vi "ex_getChanNamesFromDDT.vi"(8 "error in (no error)":errorcluster, 9 "file params":T3 {"Flags"."time preference" items=["Absolute", "Relative"]; "Flags"."x_columns" items=["None", "One", "Multiple"]; "origin time" format="%<%X\n%x>T"}, 10 "append info in":T1, 11 "Express Wave Attributes in":T2[](array[typedef]) {"dX" format="%.2f"; "X0" format="%<%X\n%x>T"; "Timestamp" format="%<%X\n%x>T"; "Start Timestamp" format="%<%X\n%x>T"}) -> (0 "error out":errorcluster, 1 "channels match":bool, 2 "channel names":string[](array[string]), 3 "Express Wave Attributes out":T2[](array[typedef]) {"dX" format="%.2f"; "X0" format="%<%X\n%x>T"; "Timestamp" format="%<%X\n%x>T"; "Start Timestamp" format="%<%X\n%x>T"}, 5 "error code":i32)   [LabVIEW 2017]
uses:
  <vilib>/express/express output/ExFileWriteBlock.llb/ex_WriteFileParams.ctl
  <vilib>/express/express input/ExFileReadBlock.llb/ex_ReadFileParams.ctl
  <vilib>/express/express shared/transition.llb/ex_WaveformAttribsPlus.ctl
  <vilib>/Platform/express/TDMExpress.llb/ex_appendInfoTDM.ctl
panel:
  out "dT":dbl[](array[numeric])
  out "Array 4":dbl[](array[numeric])
  out "channel types":string[](array[string])
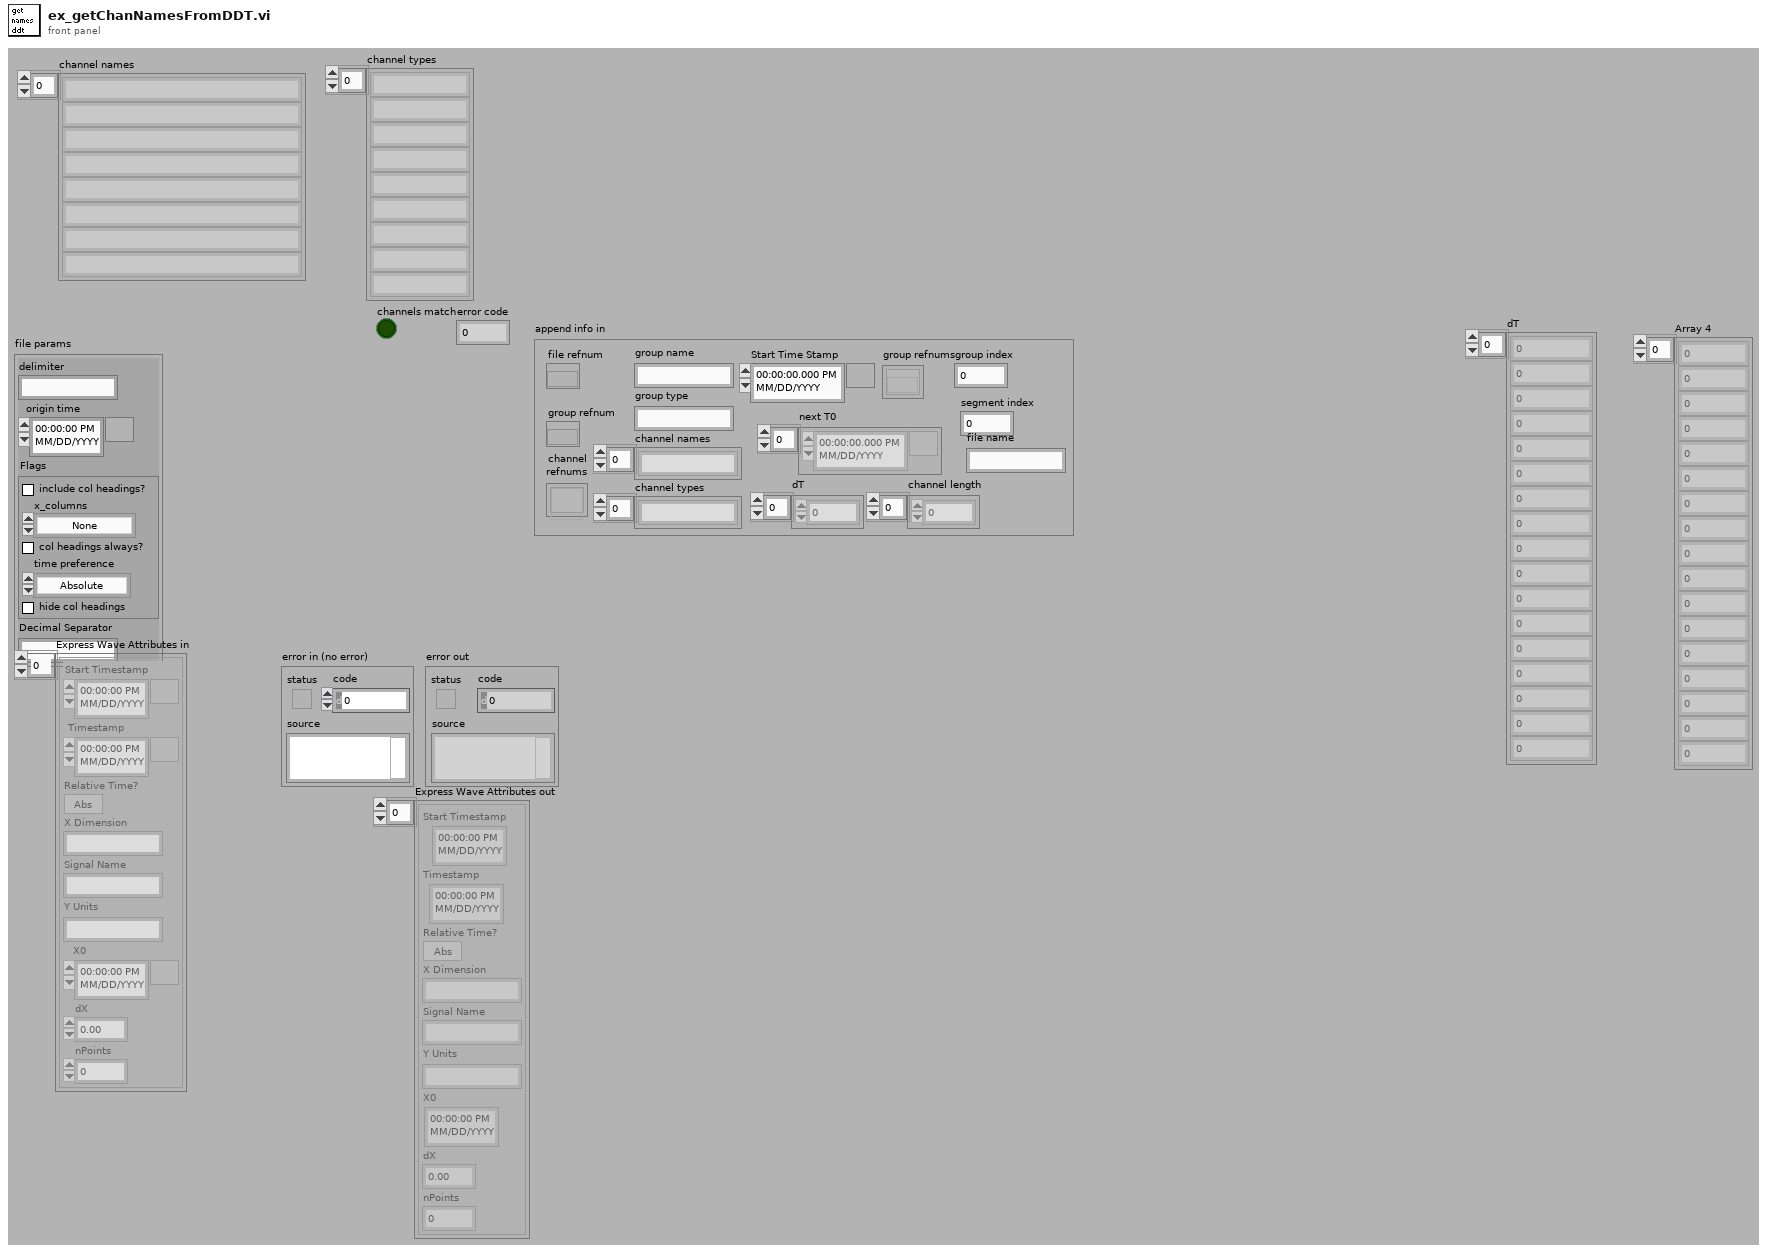
[diagram p1: front panel]
types:
  T1 = typedef "ex_appendInfoTDM.ctl" = cluster{"channel\nrefnums":refnum<k20>[], "channel names":string[], "channel types":string[], "file refnum":refnum<k20>, "group refnum":refnum<k20>, "group name":string, "group type":string, "next T0":timestamp[], "dT":dbl[], "Start Time Stamp":timestamp, "channel length":u32[], "group index":u32, "group refnums":refnum<k20>[], "file name":string, "segment index":u32}
  T2 = typedef "ex_WaveformAttribsPlus.ctl" = cluster{"Start Timestamp":timestamp, "Timestamp":timestamp, "Relative Time?":bool, "X Dimension":string, "Signal Name":string, "Y Units":string, "X0":timestamp, "dX":dbl, "nPoints":i32}
  T3 = typedef "ex_WriteFileParams.ctl" = cluster{"delimiter":string, "origin time":timestamp, "Flags":T4, "Decimal Separator":string}
  T4 = typedef "ex_ReadFileParams.ctl" = cluster{"include col headings?":bool, "x_columns":u16, "col headings always?":bool, "time preference":u16, "hide col headings":bool}
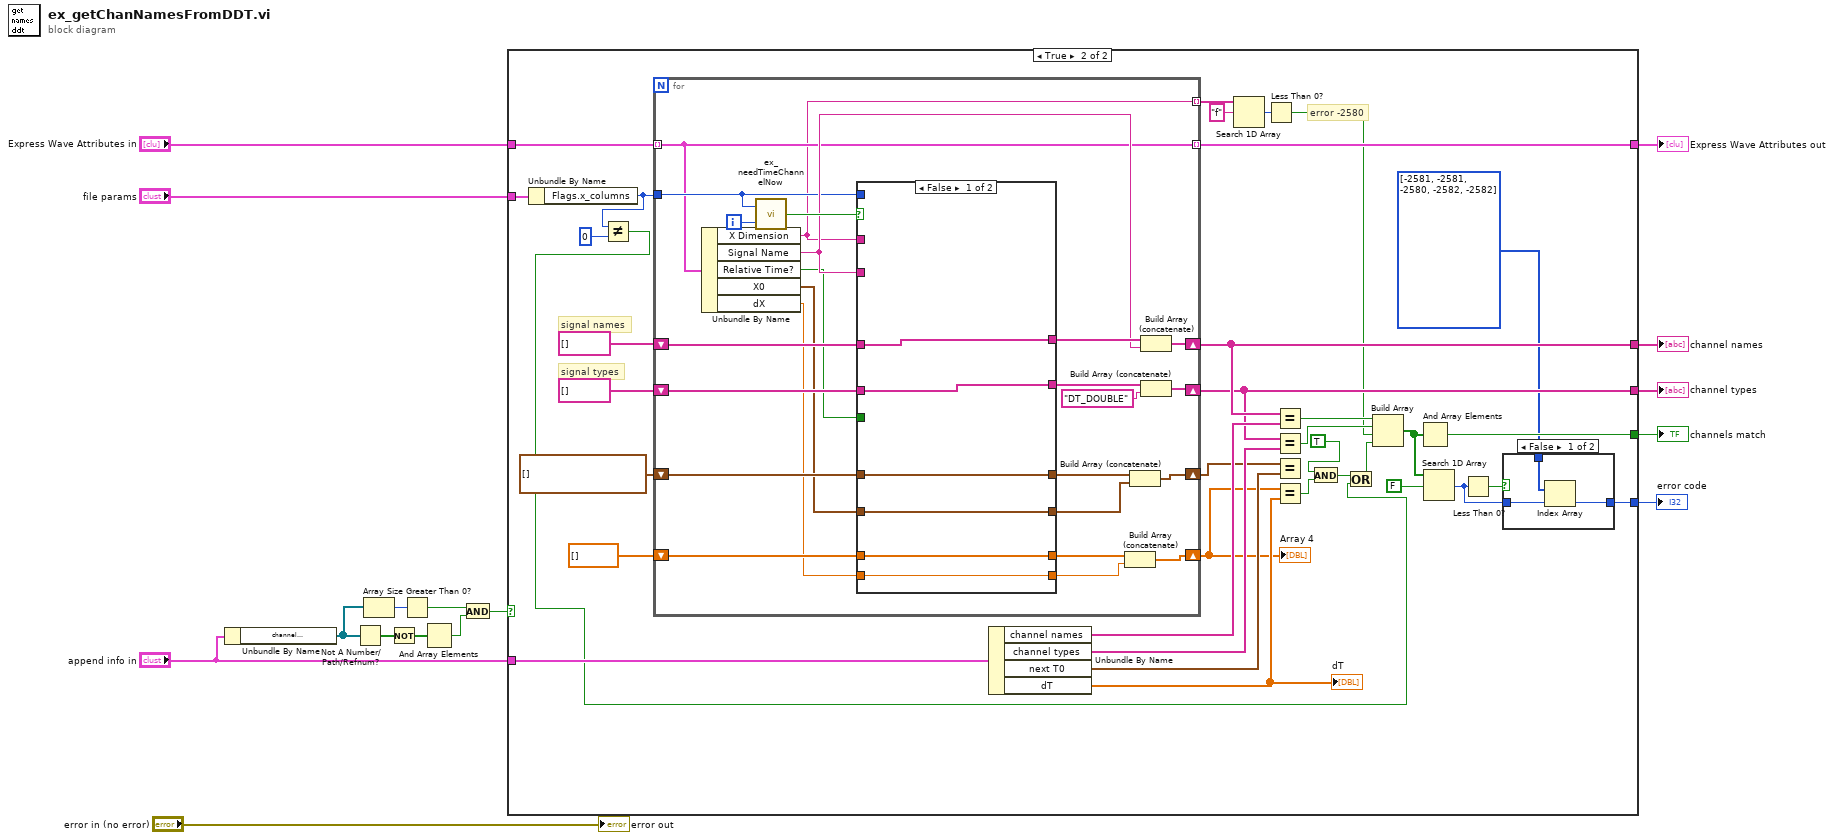
[diagram p0: block diagram]
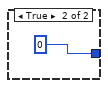
[diagram p3: hidden frame]
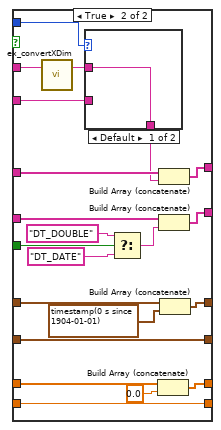
[diagram p4: hidden frame]
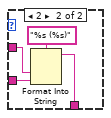
[diagram p5: hidden frame]
diagram:
  n1 = Unbundle By Name("append info in") -> ("channel\nrefnums"=w6:refnum<k20>[])
  n2 = Not A Number/Path/Refnum?(number/path/refnum=w6) -> (NaN/Path/Refnum?=w12:bool[])
  n3 = Array Size(array=w6) -> (size(s)=w5:i32)
  n4 = Not(x=w12) -> (.not. x?=w11:bool[])
  n5 = Greater Than 0?(x=w5) -> (x > 0?=w3:bool)
  n6 = And Array Elements(Boolean array=w11) -> (logical AND=w4:bool)
  n7 = And(x=w3, y=w4) -> (x .and. y?=w2:bool)
  n8 = case shown="True" w2 {
    tunnel: "file params" -> [_ w53]
    tunnel: "Express Wave Attributes in" -> [w17 w51]
    tunnel: [w17 w49] -> w13
    tunnel: [_ w48] -> w10
    tunnel: [_ w36] -> w9
    tunnel: "append info in" -> [_ w44]
    tunnel: [_ w43] -> w7
    tunnel: [_ w32] -> w1
    frame False {
    }
    frame True {
      # "error -2580"
      # "signal types"
      # "signal names"
      n9 = Unbundle By Name(w53) -> ("Flags.x_columns"=w21:u16)
      n10 = Not Equal?(x=w21, y=u16 0) -> (x != y?=w19:bool)
      n11 = for {
        tunnel: w51 -> [w69] mode=indexing
        tunnel: w21 -> [w75]
        shift-right: [w78] -> w48
        shift-left: string[] [] -> [w79]
        shift-right: [w72] -> w43
        shift-left: string[] [] -> [w74]
        tunnel: [w69] -> w49 mode=indexing
        tunnel: [w68] -> w42 mode=indexing
        shift-right: [w65] -> w26
        shift-left: timestamp[] [] -> [w67]
        shift-right: [w59] -> w25
        shift-left: dbl[] [] -> [w62]
        i -> [w81]
        n12 = Unbundle By Name(w69) -> ("X Dimension"=w68:string, "Signal Name"=w76:string, "Relative Time?"=w73:bool, "X0"=w64:timestamp, "dX"=w61:dbl)
        n13 = call <vilib>:"ex_needTimeChannelNow.vi"("index"=w81, "x_columns"=w75) -> ("need time channel NOW !!!!"=w80:bool)
        n14 = case shown="False" w80 {
          tunnel: w68 -> [_ w103]
          tunnel: w76 -> [_ w108]
          tunnel: w79 -> [w87 w107]
          tunnel: [w87 w102] -> w77
          tunnel: w75 -> [_ w105]
          tunnel: w74 -> [w86 w101]
          tunnel: w73 -> [_ w100]
          tunnel: [w86 w97] -> w71
          tunnel: w67 -> [w85 w95]
          tunnel: [w85 w94] -> w66
          tunnel: w64 -> [w84 w93]
          tunnel: [w84 w93] -> w63
          tunnel: w62 -> [w83 w91]
          tunnel: w61 -> [w82 w89]
          tunnel: [w83 w90] -> w60
          tunnel: [w82 w89] -> w58
          frame False {
          }
          frame True {
            n15 = call <vilib>:"ex_convertXDim.vi"("x_dimension in"=w103) -> ("x_dimension out"=w104:string)  [unwired: 1 in, 1 out]
            n16 = case shown="Default" w105 {
              tunnel: w104 -> [w109 w110]
              tunnel: w108 -> [_ w113]
              tunnel: [w109 w111] -> w106
              frame Default {
              }
              frame 2 {
                n17 = Format Into String(format string="%s (%s)", w110, w113) -> (resulting string=w111:string)  [unwired: 2 in, 1 out]
              }
            }
            n18 = Select(t="DT_DOUBLE", s=w100, f="DT_DATE") -> (s? t:f=w96:string)
            n19 = Build Array (concatenate)(w91, 0.0) -> (w90:dbl[])
            n20 = Build Array (concatenate)(w107, w106) -> (w102:string[])
            n21 = Build Array (concatenate)(w101, w96) -> (w97:string[])
            n22 = Build Array (concatenate)(w95, timestamp(0 s since 1904-01-01)) -> (w94:timestamp[])
          }
        }
        n23 = Build Array (concatenate)(w60, w58) -> (w59:dbl[])
        n24 = Build Array (concatenate)(w66, w63) -> (w65:timestamp[])
        n25 = Build Array (concatenate)(w77, w76) -> (w78:string[])
        n26 = Build Array (concatenate)(w71, "DT_DOUBLE") -> (w72:string[])
      }
      "Array 4" <- w25
      n27 = Unbundle By Name(w44) -> ("channel names"=w47:string[], "channel types"=w46:string[], "next T0"=w29:timestamp[], "dT"=w45:dbl[])
      "dT" <- w45
      n28 = Search 1D Array(1D array=w42, element="f") -> (index of element=w40:i32)  [unwired: 1 out]
      n29 = Less Than 0?(x=w40) -> (x < 0?=w37:bool)
      n30 = Equal?(x=w48, y=w47) -> (x = y?=w39:bool)
      n31 = Equal?(x=w43, y=w46) -> (x = y?=w38:bool)
      n32 = Equal?(x=w26, y=w29) -> ()  [unwired: 1 out]
      n33 = Equal?(x=w25, y=w45) -> (x = y?=w24:bool)
      n34 = And(x=TRUE ("element"), y=w24) -> (x .and. y?=w22:bool)
      n35 = Or(x=w22, y=w19) -> (x .or. y?=w18:bool)
      n36 = Build Array(w39, w38, w37, w18) -> (w35:bool[])
      n37 = And Array Elements(Boolean array=w35) -> (logical AND=w36:bool)
      n38 = Search 1D Array(1D array=w35, element=FALSE) -> (index of element=w31:i32)  [unwired: 1 out]
      n39 = Less Than 0?(x=w31) -> (x < 0?=w33:bool)
      n40 = case shown="False" w33 {
        tunnel: [w55 0] -> w32
        tunnel: w31 -> [w56 _]
        tunnel: i32[] [-2581, -2581, -2580, -2582, -2582] -> [w54 _]
        frame False {
          n41 = Index Array(array=w54, index=w56) -> (element=w55:i32)
        }
        frame True {
        }
      }
    }
  }
  "channel types" <- w7
  "channel names" <- w10
  "Express Wave Attributes out" <- w13
  "channels match" <- w9
  "error code" <- w1
  "error out" <- "error in (no error)"
